vi "ControlDTC.vi"(8 "error in (no error)":errorcluster, 10 "Options":T1={"Group/Type"=16777215, "Byte Lengths (KWP only)"={"Override"=FALSE, "DTC"=0, "Status"=0, "Failure"=0}} {"Group/Type" format="%.0x"}, 11 "Ref":T3) -> (0 "error out":errorcluster, 3 "Ref":T3)   [LabVIEW 2015, in "Diagnostics Host Automation API.lvlib"]
uses:
  Diagnostics Host Automation API.lvlib
  Shared/Types/HostAutomation.Ref.ctl
  <vilib>/NI/STM/TCP/TCP Connection Info.ctl
  <vilib>/NI/STM/SubVIs/MetaDataElement.ctl
  Shared/Types/DTC.Codes.ctl
  Shared/Types/Command.ControlDTC.ctl
  Shared/Types/DTC.Descriptor.Override.ctl
  <vilib>/NI/NIVS Addon Network Comm/Shared/NI VeriStand Addon Network Comm Shared.lvlib
  <vilib>/NI/STM/NI STM.lvlib
  Shared/Diagnostics Addon Shared.lvlib
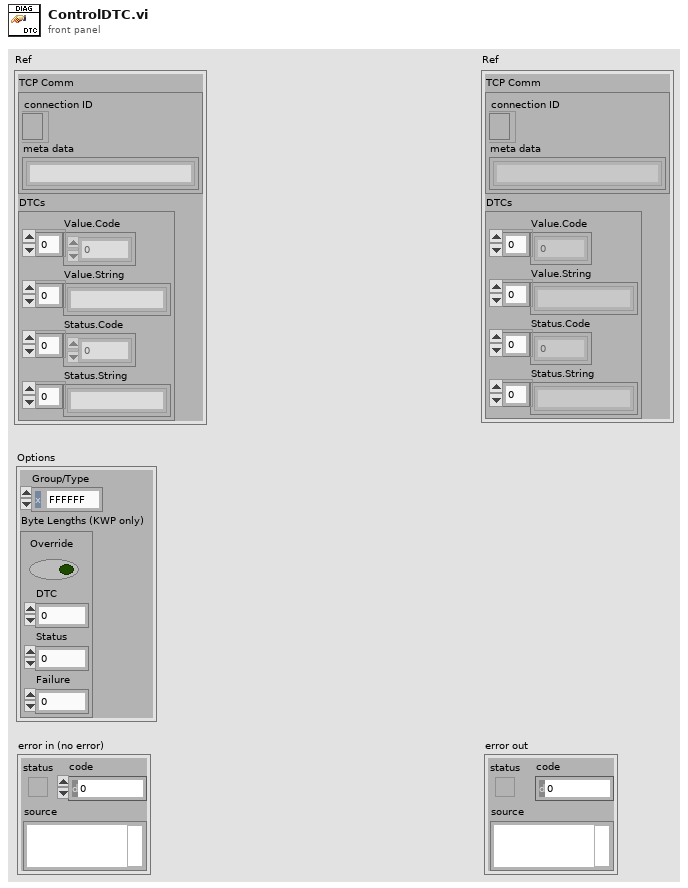
[diagram p1: front panel]
types:
  T1 = typedef "Diagnostics Addon Shared.lvlib/Command.ControlDTC.ctl" = cluster{"Group/Type":u32, "Byte Lengths (KWP only)":T2}
  T2 = typedef "Diagnostics Addon Shared.lvlib/DTC.Descriptor.Override.ctl" = cluster{"Override":bool, "DTC":u32, "Status":u32, "Failure":u32}
  T3 = typedef "Diagnostics Addon Shared.lvlib/HostAutomation.Ref.ctl" = cluster{"TCP Comm":T4, "DTCs":T6}
  T4 = typedef "NI STM.lvlib/TCP Connection Info.ctl" = cluster{"connection ID":refnum<k5>, "meta data":T5[]}
  T5 = typedef "NI STM.lvlib/MetaDataElement.ctl" = string
  T6 = typedef "Diagnostics Addon Shared.lvlib/DTC.Codes.ctl" = cluster{"Value.Code":dbl[], "Value.String":string[], "Status.Code":dbl[], "Status.String":string[]}
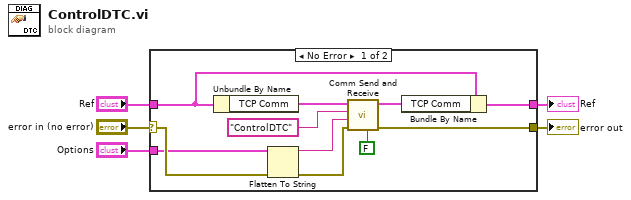
[diagram p0: block diagram]
diagram:
  n1 = case shown="No Error" "error in (no error)" {
    selector: "error in (no error)" -> [w13 w18]
    tunnel: "Ref" -> [w8 w17]
    tunnel: [w6 w17] -> w4
    tunnel: [w16 w18] -> w3
    tunnel: "Options" -> [w11 _]
    frame No Error {
      n2 = Unbundle By Name(w8) -> ("TCP Comm"=w9:T4)
      n3 = Flatten To String(anything=w11, error in (no error)=w13) -> (data string=w14:string, error out=w12:errorcluster)  [unwired: 2 in, 1 out]
      n4 = call <vilib>:"Comm Send and Receive.vi"("Resp Required?"=FALSE, "error in (no error)"=w12, "Data"=w14, "Name"="ControlDTC", "connection info"=w9) -> ("error out"=w16:errorcluster, "connection info"=w7:T4)  [unwired: 3 in, 2 out]
      n5 = Bundle By Name(cluster=w8, "TCP Comm"=w7) -> (w6:T3)
    }
    frame Error {
    }
  }
  "Ref" <- w4
  "error out" <- w3
